vi "Remove Permissions.vi"(8 "error in (no error)":errorcluster, 10 "Label":string, 11 "SQS in":refnum<class "NI_AWS_SQS.lvclass">) -> (0 "error out":errorcluster, 3 "SQS out":refnum<class "NI_AWS_SQS.lvclass">)   [LabVIEW 2015, in "NI_AWS_SQS.lvclass"]
uses:
  NI_AWS_SQS.lvclass
  Core/Name Value Pair.ctl
  Core/Request Options.ctl
  NI_AWS_SQS.lvclass/NI_AWS_SQS.ctl
  Read Account Number.vi
  Read Name.vi
  Core/NI_AWS_Core.lvclass
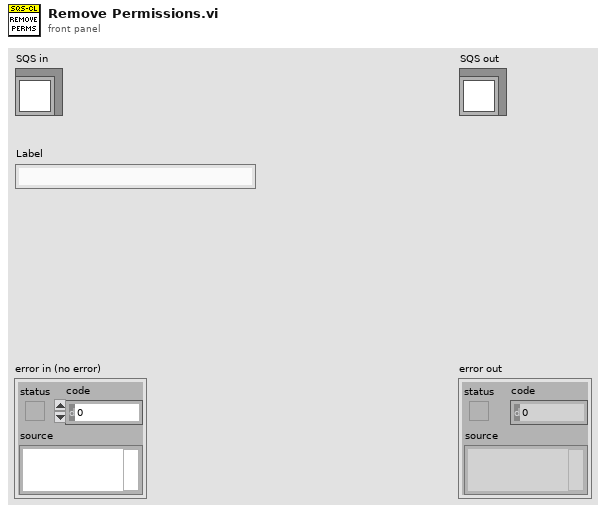
[diagram p1: front panel]
types:
  T1 = typedef "NI_AWS_Core.lvclass/Name Value Pair.ctl" = cluster{"name":string, "value":string}
  T2 = typedef "NI_AWS_Core.lvclass/Request Options.ctl" = cluster{"request headers":T1[], "request parameters":T1[], "request body":string}
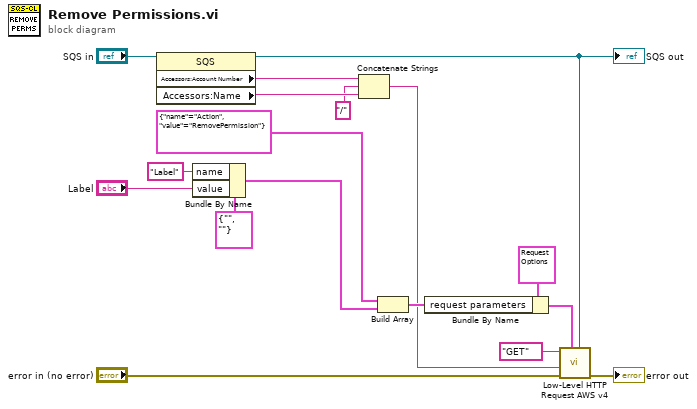
[diagram p0: block diagram]
diagram:
  n1 = property class="SQS"(reference="SQS in") -> (reference out=w9:refnum<class "NI_AWS_SQS.lvclass">, "Accessors:Account Number"=w13:string, "Accessors:Name"=w12:string)  [unwired: 1 in, 1 out]
  "SQS out" <- w9
  n2 = Bundle By Name(cluster=T1 {"name"="", "value"=""} ("element"), "name"="Label", "value"="Label") -> (w3:T1)
  n3 = Concatenate Strings(w13, "/", w12) -> (w6:string)
  n4 = Build Array(T1 {"name"="Action", "value"="RemovePermission"} ("Cluster"), w3) -> (w14:T1[])
  n5 = Bundle By Name(cluster=T2 {"request headers"=[], "request parameters"=[{"name"="Action", "value"="ListQueues"}], "request body"=""} ("Request Options"), "request parameters"=w14) -> (w15:T2)
  n6 = call "Low-Level HTTP Request AWS v4.vi"("AWS Core"=w9, "Request Options"=w15, "error in (no error)"="error in (no error)", "URL Suffix"=w6, "HTTP-Verb"="GET") -> ("error out"=→"error out":errorcluster)  [unwired: 4 in, 2 out]
